vi "Host.vi"() -> ()   [LabVIEW 2018]
uses:
  <instrlib>/niDCPower/nidcpower.llb/niDCPower Measurement Type.ctl
panel:
  in  "VLED":bool
  in  "Relay 3":bool
  in  "Relay 2":bool
  in  "Relay 1":bool
  out "Relay_3 Chart":dbl(graph)=-0.000235222149982668
  out "Relay_3_cur, A":dbl caption="measurement" format="%_6g"
  in  "Relay_3, V":dbl=6.0 caption="voltage level" format="%_6p"
  in  "Relay_3_curlim, A":dbl=0.5 caption="current limit" format="%_6p"
  in  "Период опроса, мс":u32=1
  out "Relay_2_cur, A":dbl caption="measurement" format="%_6g"
  out "Relay_2 Chart":dbl(graph)=-0.000235222149982668
  in  "Relay_2, V":dbl=6.0 caption="voltage level" format="%_6p"
  in  "Relay_2_curlim, A":dbl=0.5 caption="current limit" format="%_6p"
  in  "Стоп":bool
  in  "Питание(VCC)":bool
  in  "SEL_T, мс":u32=100
  in  "SIM_SEL":bool
  out "SEL":bool
  in  "VCC_selcur":dbl=0.02 caption="current limit" format="%_6p"
  out "VCC":i32
  out "VCC":bool
  in  "VCC, V":dbl=5.0 caption="voltage level" format="%_6p"
  in  "VCC_curlim, A":dbl=0.10000000000000003 caption="current limit" format="%_6p"
  in  "VLED_curlim, A":dbl=0.30000000000000004 caption="current limit" format="%_6p"
  out "VCC_cur, A":dbl caption="measurement" format="%_6g"
  out "VLED_cur, A":dbl caption="measurement" format="%_6g"
  in  "VLED, V":dbl=10.0 caption="voltage level" format="%_6p"
  in  "Relay_1, V":dbl=6.0 caption="voltage level" format="%_6p"
  in  "Relay_1_curlim, A":dbl=0.3 caption="current limit" format="%_6p"
  out "Relay_1_cur, A":dbl caption="measurement" format="%_6g"
  out "VLED Chart":dbl(graph)=-0.0025072983641264367
  out "Relay_1 Chart":dbl(graph)=-0.0403673797130392
  out "VCC Chart":dbl(graph)=0.17110122624002952 caption="Waveform Chart 5"
  in  "VCC/VLED":refnum<k15>="PXI1Slot2" caption="instrument handle"
  in  "Relay1/Relay2/Relay3":refnum<k15>="PXI1Slot3" caption="instrument handle"
  in  "SEL":path=path "C:/VPL/LabView_PRJ/Astrolabia_22003/SEL"
  out "Номер образца":string="0"
  # "как узнать ток через обмотку.."
  # "VCC 5 В\nток (Curlim)100мА\nпорог (selcur - single event latchup current) 20мА\nVLED 10В 300мА\nRelay 6В, посмотреть какой максимальный ток через обмотку реле с мез. \nреле кнопки реле ближе к источнику, VLED тоже"
  # "потом нужно вкулючить программу, нужна карточка\nзакоротить VCC питание посадить на землю и посмотреть, как программа с этим справимся"
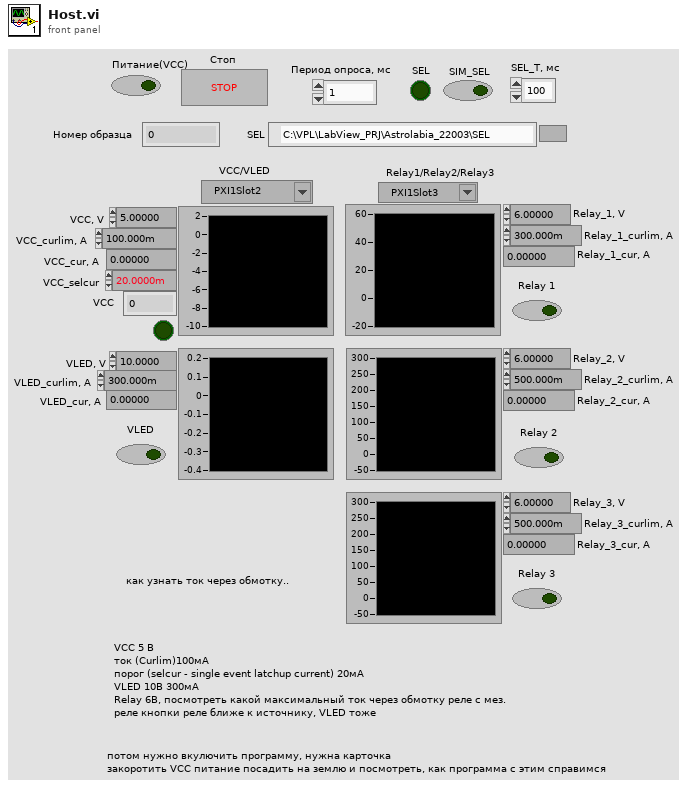
[diagram p1: front panel]
types:
  T1 = enum16{"open", "replace", "create", "open or create", "replace or create", "replace or create with confirmation"}
  T2 = typedef "niDCPower Measurement Type.ctl" = i32
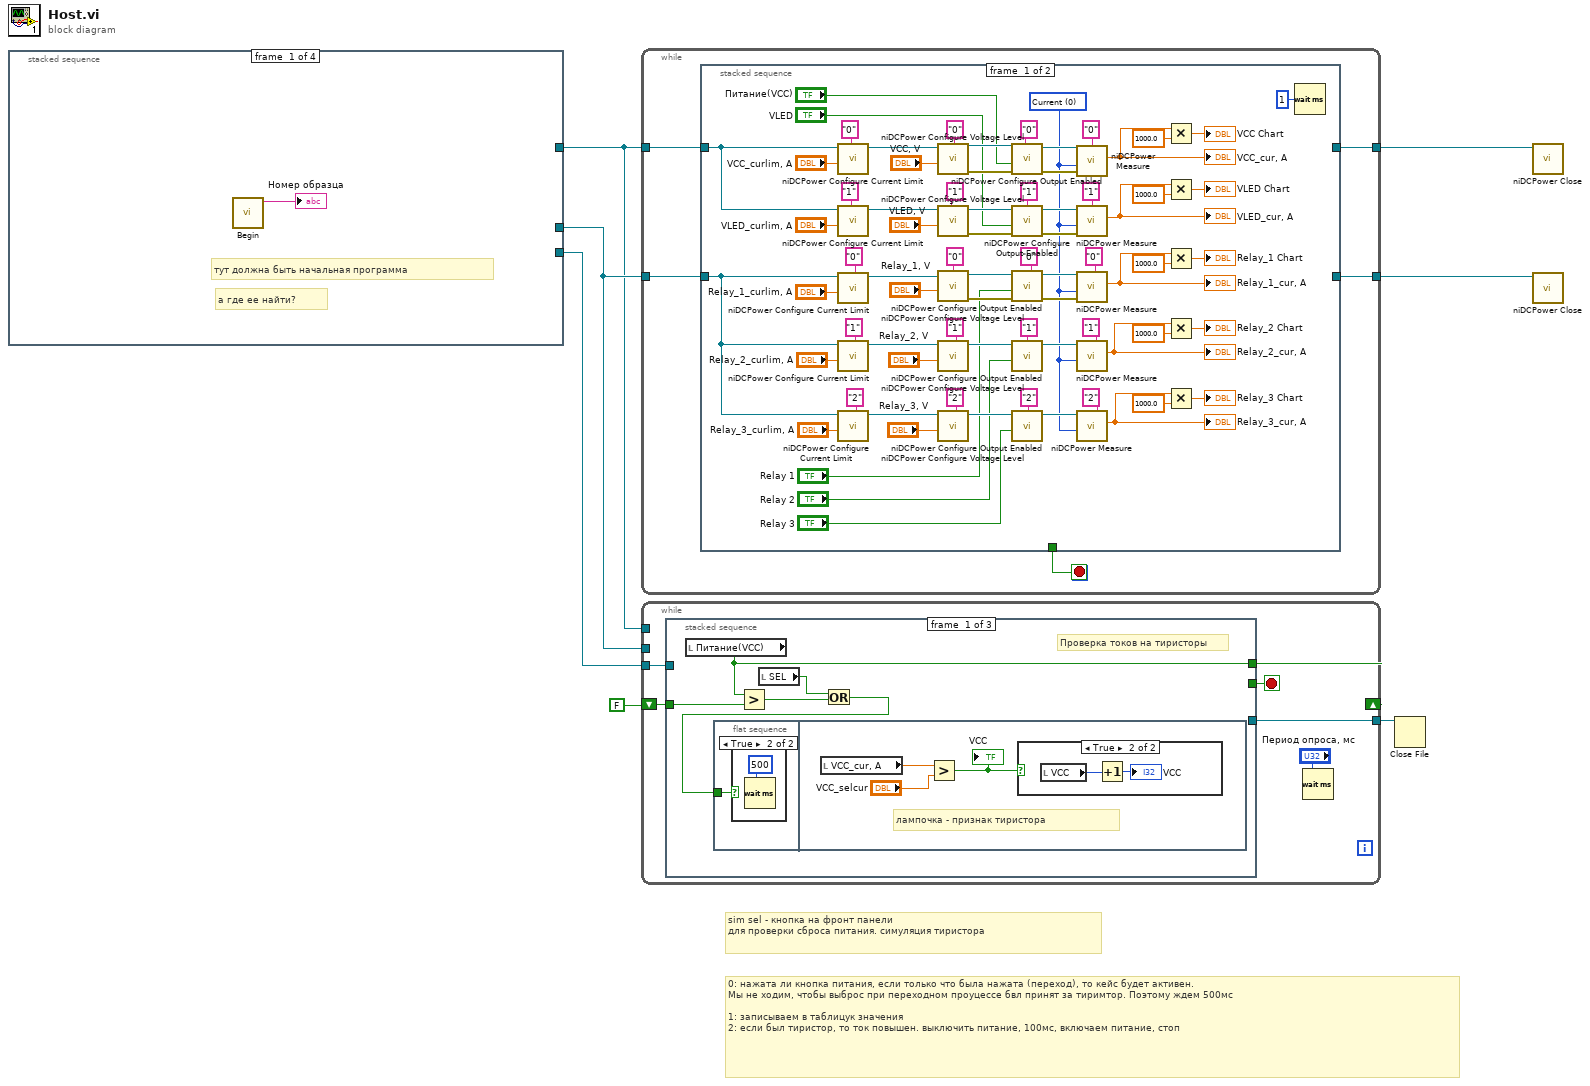
[diagram p0: block diagram]
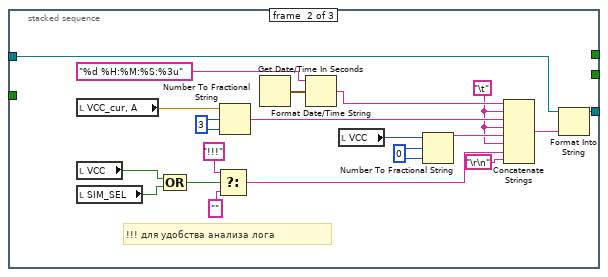
[diagram p4: hidden frame]
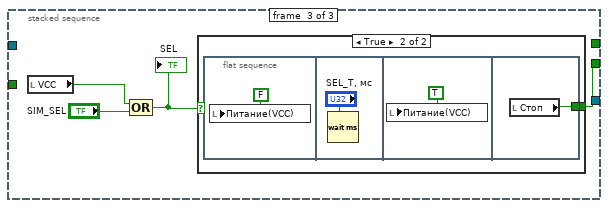
[diagram p5: hidden frame]
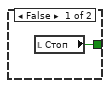
[diagram p6: hidden frame]
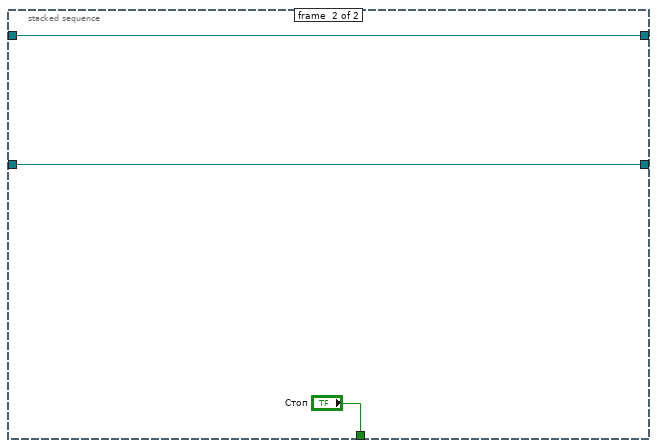
[diagram p7: hidden frame]
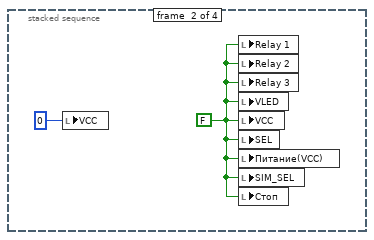
[diagram p8: hidden frame]
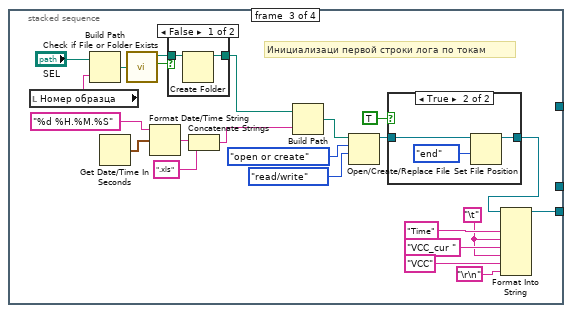
[diagram p9: hidden frame]
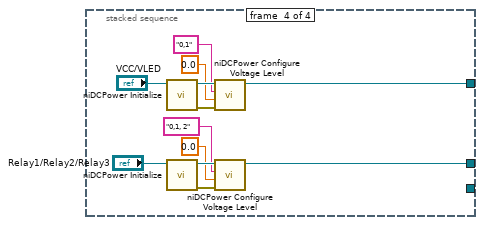
[diagram p12: hidden frame]
diagram:
  # "0: нажата ли кнопка питания, если только что была нажата (переход), то кейс будет активен. \nМы не ходим, чтобы выброс при переходном проуцессе бвл принят за тиримтор. Поэтому ждем 500мс\n\n1: записываем в таблицук значения\n2: если был тиристор, то ток повышен. выключить питание, 100мс, включаем питание, стоп"
  # "sim sel - кнопка на фронт панели\nдля проверки сброса питания. симуляция тиристора"
  n1 = stacked-sequence {
    tunnel: [_ _ _ w42] -> w4
    tunnel: [_ _ _ w41] -> w3
    tunnel: [_ _ w17 _] -> w6
    frame #0 {
      # "а где ее найти?"
      # "тут должна быть начальная программа"
      n2 = call "Begin.vi"() -> ("Номер образца 2"=→"Номер образца":string)  [unwired: 11 in]
    }
    frame #1 {
      w9 = FALSE
      n3 = local write "VCC"(0) -> ()
      n4 = local write "Relay 1"(w9) -> ()
      n5 = local write "Relay 2"(w9) -> ()
      n6 = local write "Relay 3"(w9) -> ()
      n7 = local write "VLED"(w9) -> ()
      n8 = local write "VCC"(w9) -> ()
      n9 = local write "SEL"(w9) -> ()
      n10 = local write "Питание(VCC)"(w9) -> ()
      n11 = local write "SIM_SEL"(w9) -> ()
      n12 = local write "Стоп"(w9) -> ()
    }
    frame #2 {
      w13 = "\t"
      # "Инициализаци первой строки лога по токам"
      n13 = local read "Номер образца"() -> (w29:string)
      n14 = Build Path(base path="SEL", name or relative path=w29) -> (appended path=w31:path)
      n15 = Get Date/Time In Seconds() -> (seconds since 1Jan1904=w24:timestamp)
      n16 = call <vilib>:"Check if File or Folder Exists.vi"("path"=w31) -> ("file or folder exists?"=w32:bool, "dup path"=w33:path)  [unwired: 8 in, 1 out]
      n17 = Format Date/Time String(time format string (%c)="%d %H.%M.%S", seconds (now)=w24) -> (date/time string=w21:string)  [unwired: 1 in]
      n18 = case shown="False" w32 {
        tunnel: w33 -> [w39 w40]
        tunnel: [w38 w40] -> w16
        frame False {
          n19 = Create Folder(path (use dialog)=w39) -> (created path=w38:path)  [unwired: 2 in, 2 out]
        }
        frame True {
        }
      }
      n20 = Concatenate Strings(w21, ".xls" ("string")) -> (w19:string)
      n21 = Build Path(base path=w16, name or relative path=w19) -> (appended path=w22:path)
      n22 = Open/Create/Replace File(file path (use dialog)=w22, operation (0:open)=T1."open or create", access (0:read/write)=enum16{"read/write", "read-only", "write-only"}."read/write") -> (refnum out=w25:refnum<file>)  [unwired: 3 in, 2 out]
      n23 = case shown="True" TRUE {
        tunnel: w25 -> [w34 w37]
        tunnel: [w34 w35] -> w18
        frame False {
        }
        frame True {
          n24 = Set File Position(refnum=w37, from (0:start)=enum16{"start", "end", "current"}."end") -> (refnum out=w35:refnum<file>)  [unwired: 2 in, 1 out]
        }
      }
      n25 = Format Into String(initial string=w18, "Time" ("input 1"), w13, "VCC_cur " ("input 1"), w13, "VCC" ("input 1"), "\r\n") -> (resulting string=w17:refnum<file>)  [unwired: 2 in, 1 out]
    }
    frame #3 {
      n26 = call <instrlib>:"niDCPower Initialize.vi"("resource name"="VCC/VLED") -> ("error out"=w49:errorcluster, "instrument handle out"=w51:refnum<k15>)  [unwired: 3 in, 6 out]
      n27 = call <instrlib>:"niDCPower Initialize.vi"("resource name"="Relay1/Relay2/Relay3") -> ("error out"=w50:errorcluster, "instrument handle out"=w52:refnum<k15>)  [unwired: 3 in, 6 out]
      n28 = call <instrlib>:"niDCPower Configure Voltage Level.vi"("error in (no error)"=w49, "voltage level"=0.0, "channel name"="0,1", "instrument handle"=w51) -> ("instrument handle out"=w41:refnum<k15>)  [unwired: 6 in, 1 out]
      n29 = call <instrlib>:"niDCPower Configure Voltage Level.vi"("error in (no error)"=w50, "voltage level"=0.0, "channel name"="0,1, 2", "instrument handle"=w52) -> ("instrument handle out"=w42:refnum<k15>)  [unwired: 6 in, 1 out]
    }
  }
  n30 = while {
    tunnel: w3 -> [w57]
    tunnel: w4 -> [w56]
    tunnel: [w55] -> w2
    tunnel: [w54] -> w1
    stop <- w53 stop-if-true
    n31 = stacked-sequence {
      tunnel: w56 -> [w62 w134]
      tunnel: w57 -> [w77 w135]
      tunnel: [_ w135] -> w55
      tunnel: [_ w134] -> w54
      tunnel: [_ "Стоп"] -> w53
      frame #0 {
        w63 = T2 0 items=["Current", "Voltage"] ("measurement type")
        n32 = call <instrlib>:"niDCPower Configure Current Limit.vi"("current limit"="VCC_curlim, A", "channel name"="0", "instrument handle"=w77) -> ("instrument handle out"=w121:refnum<k15>)  [unwired: 7 in, 1 out]
        n33 = call <instrlib>:"niDCPower Configure Current Limit.vi"("current limit"="VLED_curlim, A", "channel name"="1", "instrument handle"=w77) -> ("instrument handle out"=w122:refnum<k15>)  [unwired: 7 in, 1 out]
        n34 = call <instrlib>:"niDCPower Configure Current Limit.vi"("current limit"="Relay_1_curlim, A", "channel name"="0", "instrument handle"=w62) -> ("instrument handle out"=w104:refnum<k15>)  [unwired: 7 in, 1 out]
        n35 = call <instrlib>:"niDCPower Configure Current Limit.vi"("current limit"="Relay_2_curlim, A", "channel name"="1", "instrument handle"=w62) -> ("instrument handle out"=w84:refnum<k15>)  [unwired: 7 in, 1 out]
        n36 = call <instrlib>:"niDCPower Configure Current Limit.vi"("current limit"="Relay_3_curlim, A", "channel name"="2", "instrument handle"=w62) -> ("instrument handle out"=w71:refnum<k15>)  [unwired: 7 in, 1 out]
        n37 = call <instrlib>:"niDCPower Configure Voltage Level.vi"("voltage level"="VCC, V", "channel name"="0", "instrument handle"=w121) -> ("error out"=w114:errorcluster, "instrument handle out"=w117:refnum<k15>)  [unwired: 7 in]
        n38 = call <instrlib>:"niDCPower Configure Voltage Level.vi"("voltage level"="VLED, V", "channel name"="1", "instrument handle"=w122) -> ("error out"=w115:errorcluster, "instrument handle out"=w116:refnum<k15>)  [unwired: 7 in]
        n39 = call <instrlib>:"niDCPower Configure Voltage Level.vi"("voltage level"="Relay_1, V", "channel name"="0", "instrument handle"=w104) -> ("error out"=w108:errorcluster, "instrument handle out"=w109:refnum<k15>)  [unwired: 7 in]
        n40 = call <instrlib>:"niDCPower Configure Voltage Level.vi"("voltage level"="Relay_2, V", "channel name"="1", "instrument handle"=w84) -> ("instrument handle out"=w82:refnum<k15>)  [unwired: 7 in, 1 out]
        n41 = call <instrlib>:"niDCPower Configure Voltage Level.vi"("voltage level"="Relay_3, V", "channel name"="2", "instrument handle"=w71) -> ("instrument handle out"=w69:refnum<k15>)  [unwired: 7 in, 1 out]
        n42 = call <instrlib>:"niDCPower Configure Output Enabled.vi"("error in (no error)"=w114, "output enabled"="Питание(VCC)", "channel name"="0", "instrument handle"=w117) -> ("error out"=w126:errorcluster, "instrument handle out"=w125:refnum<k15>)  [unwired: 6 in]
        n43 = call <instrlib>:"niDCPower Configure Output Enabled.vi"("error in (no error)"=w115, "output enabled"="VLED", "channel name"="1", "instrument handle"=w116) -> ("error out"=w127:errorcluster, "instrument handle out"=w128:refnum<k15>)  [unwired: 6 in]
        n44 = call <instrlib>:"niDCPower Configure Output Enabled.vi"("error in (no error)"=w108, "output enabled"="Relay 1", "channel name"="0", "instrument handle"=w109) -> ("error out"=w100:errorcluster, "instrument handle out"=w101:refnum<k15>)  [unwired: 6 in]
        n45 = call <instrlib>:"niDCPower Configure Output Enabled.vi"("output enabled"="Relay 2", "channel name"="1", "instrument handle"=w82) -> ("instrument handle out"=w80:refnum<k15>)  [unwired: 7 in, 1 out]
        n46 = call <instrlib>:"niDCPower Configure Output Enabled.vi"("output enabled"="Relay 3", "channel name"="2", "instrument handle"=w69) -> ("instrument handle out"=w67:refnum<k15>)  [unwired: 7 in, 1 out]
        n47 = call <instrlib>:"niDCPower Measure.vi"("error in (no error)"=w126, "measurement type"=w63, "channel name"="0", "instrument handle"=w125) -> ("measurement"=w93:dbl)  [unwired: 5 in, 2 out]
        "VCC_cur, A" <- w93
        n48 = call <instrlib>:"niDCPower Measure.vi"("error in (no error)"=w127, "measurement type"=w63, "channel name"="1", "instrument handle"=w128) -> ("measurement"=w96:dbl)  [unwired: 5 in, 2 out]
        "VLED_cur, A" <- w96
        n49 = call <instrlib>:"niDCPower Measure.vi"("error in (no error)"=w100, "measurement type"=w63, "channel name"="0", "instrument handle"=w101) -> ("measurement"=w94:dbl)  [unwired: 5 in, 2 out]
        "Relay_1_cur, A" <- w94
        n50 = call <instrlib>:"niDCPower Measure.vi"("measurement type"=w63, "channel name"="1", "instrument handle"=w80) -> ("measurement"=w78:dbl)  [unwired: 6 in, 2 out]
        "Relay_2_cur, A" <- w78
        n51 = call <instrlib>:"niDCPower Measure.vi"("measurement type"=w63, "channel name"="2", "instrument handle"=w67) -> ("measurement"=w65:dbl)  [unwired: 6 in, 2 out]
        "Relay_3_cur, A" <- w65
        n52 = Multiply(x=w93, y=1000.0) -> (x*y=→"VCC Chart":dbl)
        n53 = Multiply(x=w96, y=1000.0) -> (x*y=→"VLED Chart":dbl)
        n54 = Multiply(x=w94, y=1000.0) -> (x*y=→"Relay_1 Chart":dbl)
        n55 = Multiply(x=w78, y=1000.0) -> (x*y=→"Relay_2 Chart":dbl)
        n56 = Multiply(x=w65, y=1000.0) -> (x*y=→"Relay_3 Chart":dbl)
        n57 = Wait (ms)(milliseconds to wait=u32 1) -> ()  [unwired: 1 out]
      }
      frame #1 {
      }
    }
  }
  n58 = while {
    shift-right: [w141] -> _
    shift-left: FALSE -> [w140]
    tunnel: w6 -> [w139]
    tunnel: [w137] -> w5
    tunnel: w4 -> [_]
    tunnel: w3 -> [_]
    stop <- w138 stop-if-true
    n59 = stacked-sequence {
      tunnel: [w145 _ _] -> w141
      tunnel: w140 -> [w146 _ _]
      tunnel: w139 -> [_ w165 _]
      tunnel: [_ _ w177] -> w138
      tunnel: [_ w164 _] -> w137
      frame #0 {
        # "Проверка токов на тиристоры"
        n60 = local read "Питание(VCC)"() -> (w145:bool)
        n61 = flat-sequence {
          tunnel: w142 -> [w147]
          frame #0 {
            n62 = case shown="True" w147 {
              frame False {
              }
              frame True {
                n63 = Wait (ms)(milliseconds to wait=u32 500) -> ()  [unwired: 1 out]
              }
            }
          }
          frame #1 {
            # "лампочка - признак тиристора"
            n64 = local read "VCC_cur, A"() -> (w149:dbl)
            n65 = Greater?(x=w149, y="VCC_selcur") -> (0:w150:bool)
            "VCC" <- w150
            n66 = case shown="True" w150 {
              frame False {
              }
              frame True {
                n67 = local read "VCC"() -> (w153:i32)
                n68 = Increment(x=w153) -> (x+1=→"VCC":i32)
              }
            }
          }
        }
        n69 = Greater?(x=w145, y=w146) -> (0:w144:bool)
        n70 = local read "SEL"() -> (w143:bool)
        n71 = Or(x=w143, y=w144) -> (x .or. y?=w142:bool)
      }
      frame #1 {
        w161 = i16 0 ("width (-)")
        w163 = i16 3 ("width (-)")
        w158 = "\t"
        # "!!! для удобства анализа лога"
        n72 = local read "VCC_cur, A"() -> (w162:dbl)
        n73 = local read "VCC"() -> (w155:bool)
        n74 = local read "SIM_SEL"() -> (w154:bool)
        n75 = Compound Arithmetic op=OR(w155, w154) -> (w166:bool)
        n76 = Select(t="!!!", s=w166, f="") -> (s? t:f=w157:string)
        n77 = Number To Fractional String(number=w162, width (-)=w163, precision (6)=w163) -> (F-format string=w167:string)  [unwired: 1 in]
        n78 = Get Date/Time In Seconds() -> (seconds since 1Jan1904=w173:timestamp)
        n79 = Format Date/Time String(time format string (%c)="%d %H:%M:%S:%3u", seconds (now)=w173) -> (date/time string=w168:string)  [unwired: 1 in]
        n80 = local read "VCC"() -> (w160:i32)
        n81 = Number To Fractional String(number=w160, width (-)=w161, precision (6)=w161) -> (F-format string=w159:string)  [unwired: 1 in]
        n82 = Concatenate Strings(w168, w158, w167, w158, w159, w158, w157, "\r\n") -> (w172:string)
        n83 = Format Into String(initial string=w165, w172) -> (resulting string=w164:refnum<file>)  [unwired: 2 in, 1 out]
      }
      frame #2 {
        n84 = local read "VCC"() -> (w175:bool)
        n85 = Compound Arithmetic op=OR(w175, "SIM_SEL") -> (w176:bool)
        "SEL" <- w176
        n86 = case shown="True" w176 {
          tunnel: [w178 w179] -> w177
          frame False {
            n87 = local read "Стоп"() -> (w178:bool)
          }
          frame True {
            n88 = flat-sequence {
              tunnel: [w183] -> w179
              frame #0 {
                n89 = local write "Питание(VCC)"(FALSE ("SYS_RESET")) -> ()
              }
              frame #1 {
                n90 = Wait (ms)(milliseconds to wait="SEL_T, мс") -> ()  [unwired: 1 out]
              }
              frame #2 {
                n91 = local write "Питание(VCC)"(TRUE ("SYS_RESET")) -> ()
              }
              frame #3 {
                n92 = local read "Стоп"() -> (w183:bool)
              }
            }
          }
        }
      }
    }
    n93 = Wait (ms)(milliseconds to wait="Период опроса, мс") -> ()  [unwired: 1 out]
  }
  n94 = Close File(refnum=w5) -> ()  [unwired: 1 in, 2 out]
  n95 = call <instrlib>:"niDCPower Close.vi"("instrument handle"=w2) -> ()  [unwired: 10 in, 1 out]
  n96 = call <instrlib>:"niDCPower Close.vi"("instrument handle"=w1) -> ()  [unwired: 10 in, 1 out]
